vi "niScope EX Fetch In Chunks.vi"() -> ()   [LabVIEW 2024]
uses:
  <instrlib>/niScope/Controls/niScope trigger source.ctl
  <instrlib>/niScope/Configure/Trigger/niScope Configure Trigger Edge.vi
  <instrlib>/niScope/Acquire/Fetch/niScope Fetch.vi
panel:
  out "# of Chunks Fetched":i32
  out "# of Points Fetched":i32
  out "Waveform":T1(graph)
  in  "Min Record Length":i32=2048
  in  "Ref. Position (%)":dbl=50.0
  in  "Min. Sample Rate":dbl=10000.0 format="%#_6p"
  in  "Vertical Range (V)":dbl=2.0 format="%_3p"
  in  "Channel":string="0"
  in  "Resource Name":refnum<k15>="Dev1" caption="Resource Name(s)"
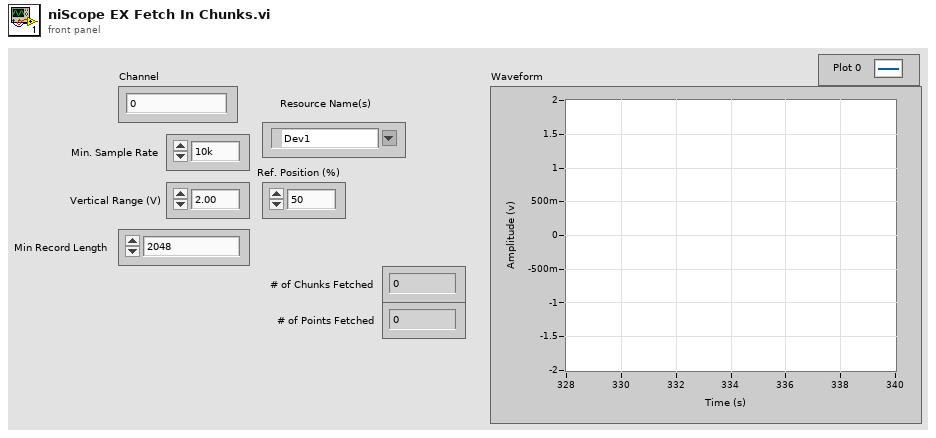
[diagram p1: front panel]
types:
  T1 = cluster{"absoluteInitialX":dbl, "xIncrement":dbl, "wfm":dbl[]}[]
  T2 = typedef "niScope trigger source.ctl" = string
  T3 = cluster{"actualSamples":i32, "absoluteInitialX":dbl, "relativeInitialX":dbl, "xIncrement":dbl, "offset":dbl, "gain":dbl, "reserved1":dbl, "reserved2":dbl}
  T4 = cluster{"absoluteInitialX":dbl, "xIncrement":dbl, "wfm":dbl[]}
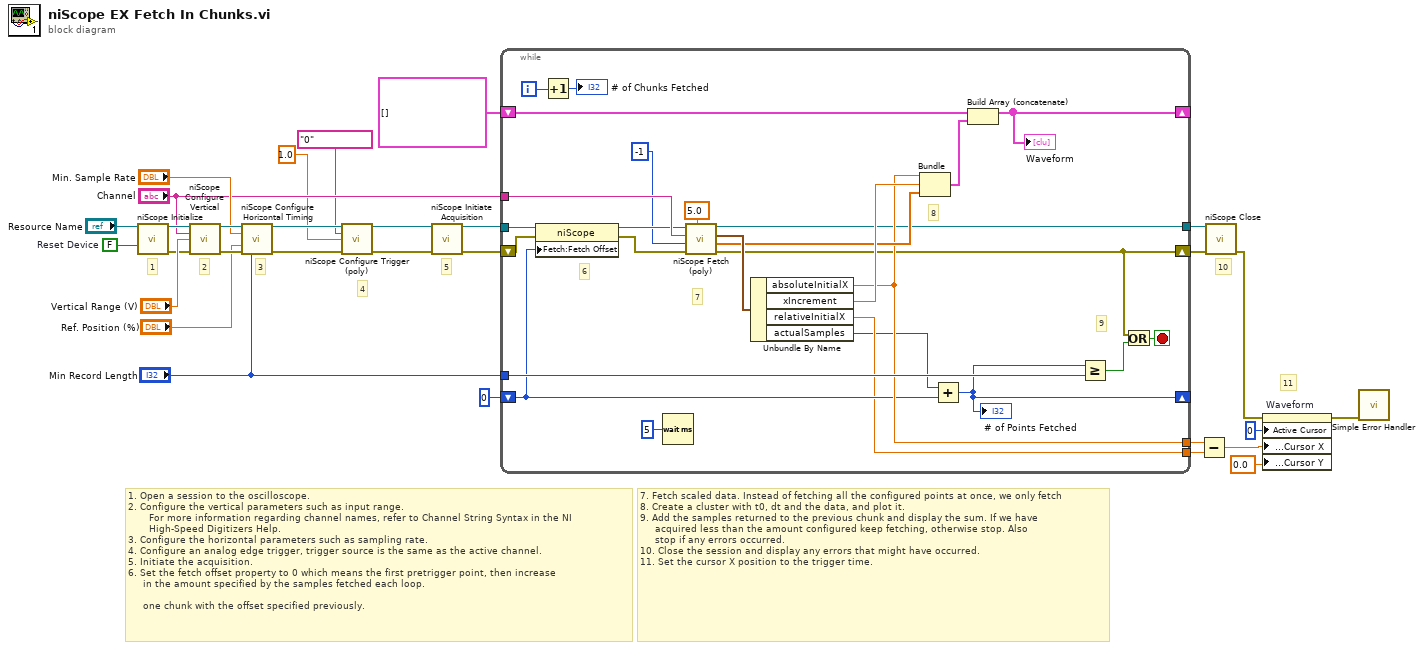
[diagram p0: block diagram]
diagram:
  w30 = FALSE  # Reset Device
  # "7. Fetch scaled data. Instead of fetching all the configured points at once, we only fetch\n8. Create a cluster with t0, dt and the data, and plot it.\n9. Add the samples returned to the previous chunk and display the sum. If we have\n     acquired less than the amount configured keep fetching, otherwise stop. Also\n     stop if any errors occurred.\n10. Close the session and display any errors that might have occurred.\n11. Set the cursor X position to the trigger time."
  # "1. Open a session to the oscilloscope.\n2. Configure the vertical parameters such as input range.\n       For more information regarding channel names, refer to Channel String Syntax in the NI            \n       High-Speed Digitizers Help.\n3. Configure the horizontal parameters such as sampling rate.\n4. Configure an analog edge trigger, trigger source is the same as the active channel.\n5. Initiate the acquisition.\n6. Set the fetch offset property to 0 which means the first pretrigger point, then increase\n     in the amount specified by the samples fetched each loop.\n\n     one chunk with the offset specified previously."
  # "11"
  # "10"
  # "5"
  # "4"
  # "3"
  # "2"
  # "1"
  n1 = call <instrlib>:"niScope Initialize.vi"("resource name"="Resource Name", "reset device"=w30) -> ("instrument handle"=w20:refnum<k15>, "error out"=w19:errorcluster)  [unwired: 12 in]
  n2 = call <instrlib>:"niScope Configure Vertical.vi"("instrument handle"=w20, "channels"="Channel", "vertical range"="Vertical Range (V)", "error in"=w19) -> ("instrument handle out"=w27:refnum<k15>, "error out"=w28:errorcluster)  [unwired: 10 in]
  n3 = call <instrlib>:"niScope Configure Horizontal Timing.vi"("instrument handle"=w27, "min sample rate"="Min. Sample Rate", "reference position"="Ref. Position (%)", "error in"=w28, "min record length"="Min Record Length") -> ("instrument handle out"=w14:refnum<k15>, "error out"=w13:errorcluster)  [unwired: 9 in]
  n4 = call-poly <instrlib>:"niScope Configure Trigger (poly).vi"("instrument handle"=w14, "trigger source"=T2 "0", "trigger level"=1.0, "error in"=w13) -> ("instrument handle out"=w12:refnum<k15>, "error out"=w11:errorcluster)  [unwired: 10 in]
  n5 = call <instrlib>:"niScope Initiate Acquisition.vi"("instrument handle"=w12, "error in"=w11) -> ("instrument handle out"=w7:refnum<k15>, "error out"=w6:errorcluster)  [unwired: 12 in]
  n6 = while {
    tunnel: [w35] -> w16
    tunnel: [w46] -> w17
    tunnel: "Min Record Length" -> [w54]
    shift-left: 0 -> [w38]
    shift-right: [w44] -> _
    shift-left: T1 [] -> [w56]
    shift-right: [w55] -> _
    tunnel: "Channel" -> [w50]
    tunnel: w7 -> [w40]
    tunnel: [w42] -> w9
    shift-right: [w32] -> w8
    shift-left: w6 -> [w39]
    i -> [w52]
    stop <- w53 stop-if-true
    # "6"
    # "9"
    # "8"
    # "7"
    n7 = property class="niScope"(reference=w40, error in=w39, "Fetch:Fetch Offset"=w38) -> (reference out=w37:refnum<k15>, error out=w36:errorcluster)
    n8 = Increment(x=w52) -> (x+1=→"# of Chunks Fetched":i32)
    n9 = Wait (ms)(milliseconds to wait=u32 5) -> ()  [unwired: 1 out]
    n10 = call-poly <instrlib>:"niScope Fetch (poly).vi"("timeout"=5.0, "error in"=w36, "numSamples"=-1, "channels"=w50, "instrument handle"=w37) -> ("error out"=w32:errorcluster, "wfm"=w47:dbl[], "wfm info"=w49:T3, "instrument handle out"=w42:refnum<k15>)  [unwired: 3 in]
    n11 = Unbundle By Name(w49) -> ("absoluteInitialX"=w46:dbl, "xIncrement"=w48:dbl, "relativeInitialX"=w35:dbl, "actualSamples"=w34:i32)
    n12 = Bundle("absoluteInitialX"=w46, "xIncrement"=w48, "wfm"=w47) -> (w45:T4)  [unwired: 1 in]
    n13 = Add(x=w34, y=w38) -> (x+y=w44:i32)
    "# of Points Fetched" <- w44
    n14 = Build Array (concatenate)(w56, w45) -> (w55:T1)
    "Waveform" <- w55
    n15 = Greater Or Equal?(x=w44, y=w54) -> (x >= y?=w43:bool)
    n16 = Or(x=w32, y=w43) -> (x .or. y?=w53:bool)
  }
  n17 = Subtract(x=w17, y=w16) -> (x-y=w18:dbl)
  n18 = call <instrlib>:"niScope Close.vi"("instrument handle"=w9, "error in"=w8) -> ("error out"=w4:errorcluster)  [unwired: 13 in]
  n19 = property on="Waveform" class="WFGraph (strict)"(error in=w4, "Active Cursor"=u32 0 ("Write Attribute"), "Cursor.Cursor Position:Cursor X"=w18, "Cursor.Cursor Position:Cursor Y"=0.0 ("Write Attribute")) -> (error out=w3:errorcluster)  [unwired: 1 in, 1 out]
  n20 = call <vilib>:"Simple Error Handler.vi"("error in (no error)"=w3) -> ()  [unwired: 4 in, 5 out]
